vi "Write ConvBox Handler.vi"(8 "error in (no error)":errorcluster, 9 "Data Length":string, 10 "Data":string, 11 "Listener in":refnum<class "Listener.lvclass">) -> (0 "error out":errorcluster, 3 "Listener out":refnum<class "Listener.lvclass">)   [LabVIEW 2019, in "Listener.lvclass"]
uses:
  Listener.lvclass
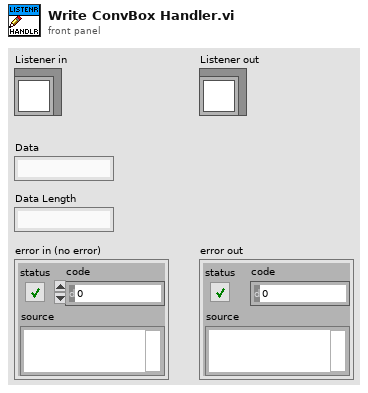
[diagram p1: front panel]
types:
  T1 = typedef "Listener.lvclass/RS-xxx To GPIB ConvBox Data Structure.ctl" = cluster{"Protocol Port Ref":refnum<visa-resource-name>, "Listener Port Ref":refnum<visa-resource-name>, "Data":string, "Command Messages Read":string[], "Address":string}
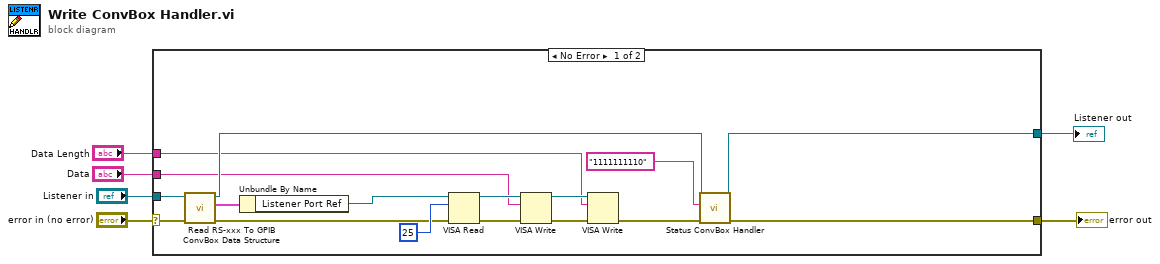
[diagram p0: block diagram]
diagram:
  n1 = case shown="No Error" "error in (no error)" {
    selector: "error in (no error)" -> [w19 w25]
    tunnel: [w15 w25] -> w6
    tunnel: "Data" -> [w13 _]
    tunnel: "Data Length" -> [w8 _]
    tunnel: "Listener in" -> [w20 w24]
    tunnel: [w16 w24] -> w1
    frame No Error {
      n2 = call-dynamic "Read RS-xxx To GPIB ConvBox Data Structure.vi"("error in (no error)"=w19, "Listener in"=w20) -> ("error out"=w12:errorcluster, "RS-xxx To GPIB ConvBox Data Structure"=w18:T1, "Listener out"=w17:refnum<class "Listener.lvclass">)  [unwired: 7 in]
      n3 = Unbundle By Name(w18) -> ("Listener Port Ref"=w7:refnum<visa-resource-name>)
      n4 = VISA Read(VISA resource name=w7, byte count=u32 25, error in (no error)=w12) -> (VISA resource name out=w23:refnum<visa-resource-name>, error out=w22:errorcluster)  [unwired: 2 out]
      n5 = VISA Write(VISA resource name=w23, write buffer=w13, error in (no error)=w22) -> (VISA resource name out=w11:refnum<visa-resource-name>, error out=w10:errorcluster)  [unwired: 1 out]
      n6 = VISA Write(VISA resource name=w11, write buffer=w8, error in (no error)=w10) -> (error out=w9:errorcluster)  [unwired: 2 out]
      n7 = call "Status ConvBox Handler.vi"("error in(no error)"=w9, "Value In"="1111111110" ("write buffer"), "Listener in"=w17) -> ("error out"=w15:errorcluster, "Listener out"=w16:refnum<class "Listener.lvclass">)  [unwired: 7 in]
    }
    frame Error {
    }
  }
  "error out" <- w6
  "Listener out" <- w1
